vi "Construct.vi"(8 "error in":errorcluster, 9 "logging configuration":T1, 10 "hardware configuration file on target":path, 11 "device parameters":T3) -> (0 "error out":errorcluster, 3 "Ballard ARINC-429 shared resources out":refnum<class "Shared Resources.lvclass">)   [LabVIEW 2020, in "Ballard ARINC 429 Engine.lvlib" / "Implementation.lvlib" / "Shared Resources.lvclass"]
uses:
  Shared Resources.lvclass
  Shared/Device Parameters.ctl
  Shared/Initialization Method.ctl
  Custom Device/Logging Configuration.ctl
  Shared/Data Word Format.ctl
  Shared Resources.lvclass/Shared Resources.ctl
  Custom Device/Custom Device.lvlib
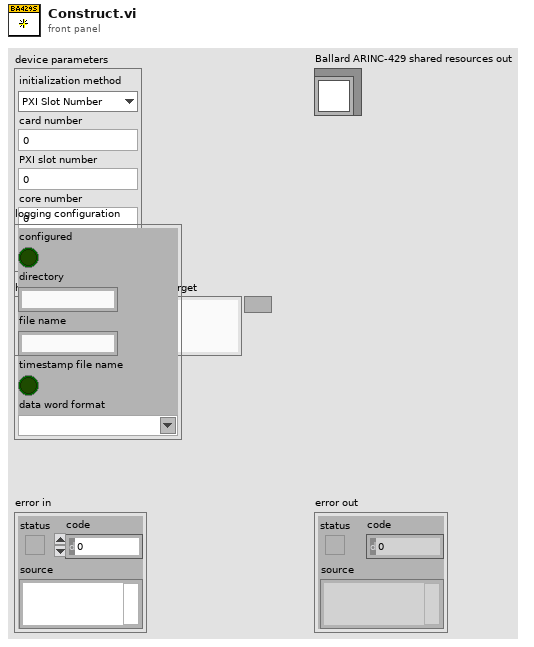
[diagram p1: front panel]
types:
  T1 = typedef "Ballard ARINC 429 Engine.lvlib/Custom Device.lvlib/Logging Configuration.ctl" = cluster{"configured":bool, "directory":string, "file name":string, "timestamp file name":bool, "data word format":T2}
  T2 = typedef "Data Word Format.ctl" = string
  T3 = typedef "Device Parameters.ctl" = cluster{"initialization method":T4, "card number":i32, "PXI slot number":i32, "core number":i32, "core serial number":i32}
  T4 = typedef "Initialization Method.ctl" = enum16{"PXI Slot Number", "Card Number", "Core Serial Number"}
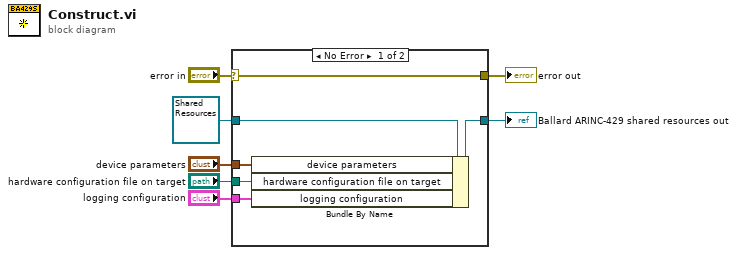
[diagram p0: block diagram]
diagram:
  n1 = case shown="No Error" "error in" {
    selector: "error in" -> [w13 w15]
    tunnel: [w13 w15] -> w6
    tunnel: [w9 w14] -> w5
    tunnel: refnum<class "Shared Resources.lvclass"> refnum ("Ballard ARINC-429 Shared Resources out") -> [w12 w14]
    tunnel: "device parameters" -> [w11 _]
    tunnel: "hardware configuration file on target" -> [w10 _]
    tunnel: "logging configuration" -> [w8 _]
    frame No Error {
      n2 = Bundle By Name(cluster=w12, "device parameters"=w11, "hardware configuration file on target"=w10, "logging configuration"=w8) -> (w9:refnum<class "Shared Resources.lvclass">)
    }
    frame Error {
    }
  }
  "error out" <- w6
  "Ballard ARINC-429 shared resources out" <- w5
